vi "Test Process within App Log Error Message.vi"(8 "error in (no error)":errorcluster, 11 "Test Case In":refnum<class "Logger Test.lvclass">) -> (0 "error out":errorcluster, 3 "Test Case Out":refnum<class "Logger Test.lvclass">)   [LabVIEW 2020, in "Logger Test.lvclass"]
uses:
  Logger Test.lvclass
  C:/Program Files (x86)/National Instruments/LabVIEW 2020/vi.lib/Astemes/LUnit/Test Case.lvclass
  source/Framework Test Suite/Mock Log Handler/Mock Log Handler.lvclass
  C:/Git/astemes-triarc-framework/source/Framework/Logging/Logging.lvclass
  source/Framework/Application/Application.lvclass
  C:/Git/astemes-triarc-framework/source/Framework/Process/Process.lvclass
  source/Framework Test Suite/Mock Process/Mock Process.lvclass
  source/Framework/Process/Process.lvclass/Process.ctl
  source/Framework/Application/Application.lvclass/Application.ctl
  <vilib>/Astemes/LUnit/Test Case.lvclass/Test Case.ctl
  <vilib>/Astemes/LUnit/LUnit Assertion Result.lvclass/LUnit Assertion Result.ctl
  <vilib>/Astemes/LUnit/LUnit Test Case Result.lvclass/LUnit Test Case Result.ctl
  <vilib>/Astemes/LUnit/LUnit Method Result.lvclass/LUnit Method Result.ctl
  source/Framework/Process/Public/Lifecycle/Get Lifecycle State.vi
  source/Framework/Process/Protected/Messaging/Enqueue Message.vi
  source/Framework/Application/Private/Add Process to Map.vi
  source/Framework/Application/Private/Start Idle Processes if Running.vi
  source/Framework/Application/Private/Throw Error If Process Already in App.vi
  source/Framework/Process/Protected/SubVIs/Set Context.vi
  source/Framework/Process/Private/SubVIs/Wait for finish.vi
  source/Framework/Process/Private/SubVIs/Set Lifecycle State.vi
  <vilib>/Astemes/LUnit/Palette/Pass If Equal.vi/cbf50e99-f124-4847-863a-8e9794d3dede.vi
  source/Framework/Process/Private/SubVIs/Handle Debug Data.vi
  source/Framework/Application/Public/Get Process.vi
  source/Framework/Process/Public/Lifecycle/Leave Process Loop.vi
  <vilib>/Astemes/LUnit/Palette/Pass.vi
  <vilib>/Astemes/LUnit/Palette/Fail.vi
  <vilib>/Astemes/LUnit/Compare Variants.vi
  <vilib>/Astemes/LUnit/Describe Comparison.vi
  <vilib>/Astemes/LUnit/Set Assertion Type.vi
  source/Framework/Logging/Log Debug.vi
  <vilib>/AdvancedString/1D String Array to Delimited String.vi
  <vilib>/Utility/High Resolution Relative Seconds.vi
  source/Framework/Application/Private/Retrieve Process from App.vi
  source/Framework/Application/Private/Parse Process Name.vi
  source/Framework/Application/Private/Get Process from Map.vi
  <vilib>/Astemes/LUnit/Add test result.vi
  <vilib>/Astemes/LUnit/LUnit Write Passed.vi
  <vilib>/Astemes/LUnit/LUnit Write Message.vi
  <vilib>/Astemes/LUnit/LUnit Write Description.vi
  <vilib>/Astemes/LUnit/Variant to string.vi
  <vilib>/Astemes/LUnit/LUnit Write Assertion Type.vi
  source/Framework/Process/Protected/Messaging/Request Message.vi
  <vilib>/AdvancedString/Delimited String to 1D String Array.vi
  <vilib>/Astemes/LUnit/LUnit Record Assertion Result.vi
  source/Framework/Process/Private/SubVIs/Enqueue Request Message.vi
  <vilib>/Astemes/LUnit/LUnit Aggregate Assertion Results.vi
  <vilib>/Astemes/LUnit/Assertion Result/LUnit Read Status.vi
  <vilib>/Astemes/LUnit/LUnit Read Message.vi
  <vilib>/Astemes/LUnit/LUnit Read Description.vi
  <vilib>/Astemes/LUnit/Method Result/LUnit Merge Status.vi
  <vilib>/Astemes/LUnit/LUnit Concatenate result strings.vi
  <vilib>/Utility/error.llb/Error Cluster From Error Code.vi
  source/Framework/Process/Public/Read Name.vi
  source/Framework/Process/Private/SubVIs/Wait for Response Message.vi
  <vilib>/Utility/Data Type/Get Type Information.vi
  <vilib>/Utility/LVClass/Get LV Class Name.vi
  source/Framework/Process/Process.lvclass
  <vilib>/Astemes/LUnit/LUnit Assertion Result.lvclass
  source/Framework/Logging/Logging.lvclass
  Logger Test.lvclass/Logger Test.ctl
  <vilib>/Astemes/LUnit/Test Case.lvclass
  source/Framework Test Suite/Support/Framework Test Support.lvlib
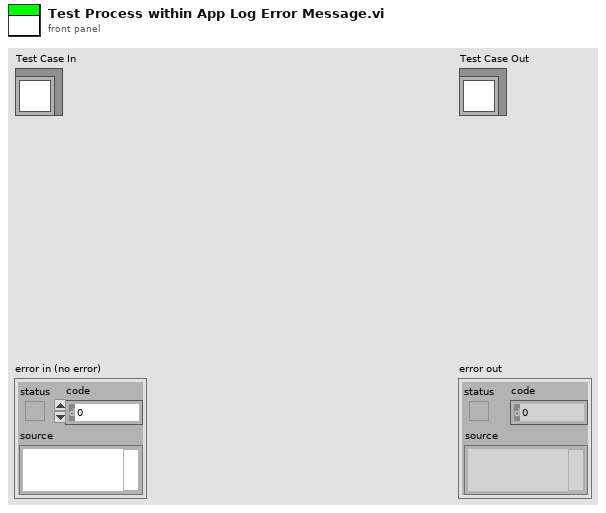
[diagram p1: front panel]
types:
  T1 = typedef "Mock Log Handler.lvclass/Log Entry.ctl" = cluster{"Level":string, "Source":string, "Message":string}
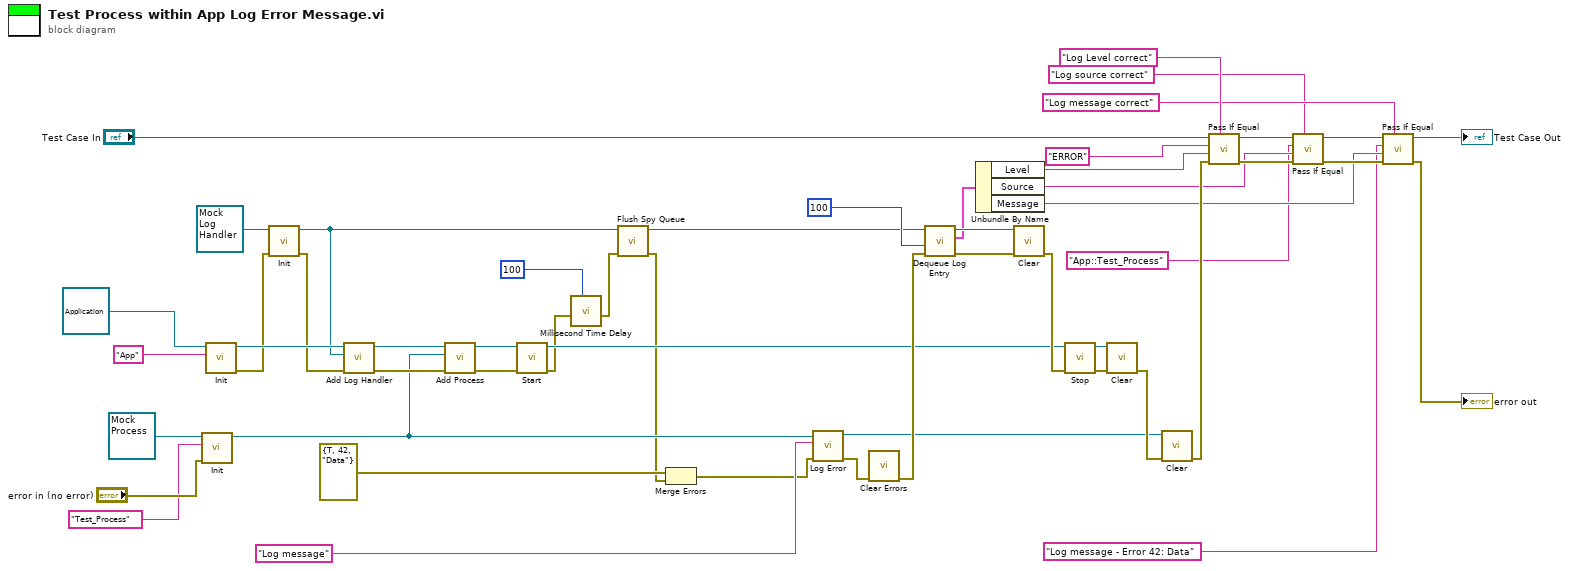
[diagram p0: block diagram]
diagram:
  n1 = call-dynamic "Init.vi"("error in (no error)"="error in (no error)", "Name"="Test_Process", "Mock Process In"=refnum<class "Mock Process.lvclass"> refnum) -> ("Mock Process Out"=w3:refnum<class "Mock Process.lvclass">)  [unwired: 7 in, 1 out]
  n2 = call-dynamic "Init.vi"("Name"="App", "Process In"=refnum<class "Application.lvclass"> refnum ("Application.lvclass")) -> ("error out"=w46:errorcluster, "Process Out"=w49:refnum<class "Application.lvclass">)  [unwired: 8 in]
  n3 = call-dynamic "Init.vi"("error in (no error)"=w46, "Mock Log Handler In"=refnum<class "Mock Log Handler.lvclass"> refnum ("Mock Log Handler.lvclass")) -> ("error out"=w45:errorcluster, "Mock Log Handler Out"=w9:refnum<class "Mock Log Handler.lvclass">)  [unwired: 8 in]
  n4 = call "Add Log Handler.vi"("error in (no error)"=w45, "Log Handler"=w9, "Process In"=w49) -> ("error out"=w19:errorcluster, "Process Out"=w18:refnum<class "Application.lvclass">)  [unwired: 7 in]
  n5 = call "Add Process.vi"("error in (no error)"=w19, "Process"=w3, "Application In"=w18) -> ("error out"=w15:errorcluster, "Application Out"=w4:refnum<class "Application.lvclass">)  [unwired: 7 in]
  n6 = call "Start.vi"("error in (no error)"=w15, "Process In"=w4) -> ("error out"=w7:errorcluster, "Process Out"=w11:refnum<class "Application.lvclass">)  [unwired: 7 in, 1 out]
  n7 = call "Millisecond Time Delay.vi"("milliseconds to wait"=u32 100, "error in (no error)"=w7) -> ("error out"=w6:errorcluster)  [unwired: 7 in]
  n8 = call "Flush Spy Queue.vi"("error in (no error)"=w6, "Mock Log Handler in"=w9) -> ("error out"=w1:errorcluster, "Mock Log Handler out"=w8:refnum<class "Mock Log Handler.lvclass">)  [unwired: 7 in, 1 out]
  n9 = Merge Errors(errorcluster {"status"=TRUE, "code"=42, "source"="Data"} ("error in (no error)"), w1) -> (w2:errorcluster)
  n10 = call "Log Error.vi"("error in (no error)"=w2, "Message"="Log message", "Logging In"=w3) -> ("error out"=w25:errorcluster, "Logging Out"=w12:refnum<class "Mock Process.lvclass">)  [unwired: 7 in]
  n11 = call <vilib>:"Clear Errors.vi"("error in (no error)"=w25) -> ("error out"=w24:errorcluster)  [unwired: 5 in, 1 out]
  n12 = call "Dequeue Log Entry.vi"("error in (no error)"=w24, "timeout in ms (-1)"=100, "Mock Log Handler in"=w8) -> ("error out"=w43:errorcluster, "Entry"=w40:T1, "Mock Log Handler out"=w44:refnum<class "Mock Log Handler.lvclass">)  [unwired: 5 in, 1 out]
  n13 = Unbundle By Name(w40) -> ("Level"=w39:string, "Source"=w29:string, "Message"=w28:string)
  n14 = call-dynamic "Clear.vi"("error in (no error)"=w43, "Mock Log Handler In"=w44) -> ("error out"=w41:errorcluster)  [unwired: 9 in]
  n15 = call "Stop.vi"("error in (no error)"=w41, "Process In"=w11) -> ("error out"=w14:errorcluster, "Process Out"=w13:refnum<class "Application.lvclass">)  [unwired: 7 in, 1 out]
  n16 = call-dynamic "Clear.vi"("error in (no error)"=w14, "Application In"=w13) -> ("error out"=w48:errorcluster)  [unwired: 9 in]
  n17 = call-dynamic "Clear.vi"("error in (no error)"=w48, "Mock Process In"=w12) -> ("error out"=w33:errorcluster)  [unwired: 9 in]
  n18 = call <vilib>:"Pass If Equal.vi"("Description"="Log Level correct", "error in (no error)"=w33, "Actual"=w39, "Expected"="ERROR", "LUnit Test Case In"="Test Case In") -> ("error out"=w35:errorcluster, "LUnit Test Case Out"=w51:refnum<class "Logger Test.lvclass">)  [unwired: 5 in]
  n19 = call <vilib>:"Pass If Equal.vi"("Description"="Log source correct", "error in (no error)"=w35, "Actual"=w29, "Expected"="App::Test_Process" ("Name"), "LUnit Test Case In"=w51) -> ("error out"=w34:errorcluster, "LUnit Test Case Out"=w37:refnum<class "Logger Test.lvclass">)  [unwired: 5 in]
  n20 = call <vilib>:"Pass If Equal.vi"("Description"="Log message correct", "error in (no error)"=w34, "Actual"=w28, "Expected"="Log message - Error 42: Data" ("Message"), "LUnit Test Case In"=w37) -> ("error out"=→"error out":errorcluster, "LUnit Test Case Out"=→"Test Case Out":refnum<class "Logger Test.lvclass">)  [unwired: 5 in]
